vi "clean up vis blockdiagram.vi"(8 "error in (no error)":errorcluster, 10 "Cleanup VI Argument":T3, 11 "Data Cluster in":T1) -> (0 "error out":errorcluster, 2 "Cleanup VI (Reply Payload)":T2, 3 "Data Cluster out":T1)   [LabVIEW 2025, in "Scripting Server.lvlib"]
uses:
  Scripting Server.lvlib
  Cleanup VI Argument--cluster.ctl
  Cleanup VI (Reply Payload)--cluster.ctl
  Module Data--cluster.ctl
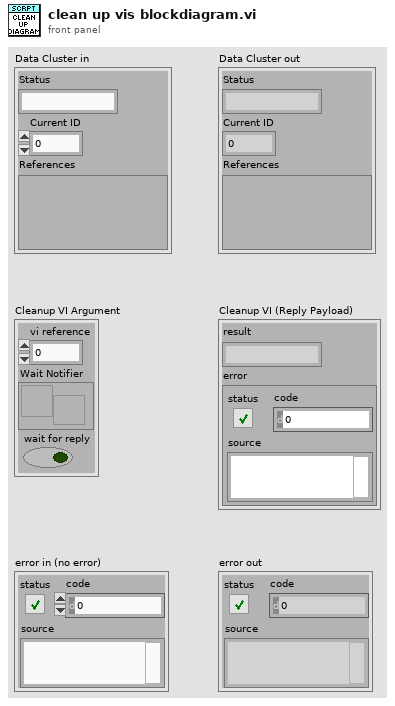
[diagram p1: front panel]
types:
  T1 = typedef "Scripting Server.lvlib/Module Data--cluster.ctl" = cluster{"Status":string, "Current ID":i32, "References":variant}
  T2 = typedef "Scripting Server.lvlib/Cleanup VI (Reply Payload)--cluster.ctl" = cluster{"result":string, "error":errorcluster}
  T3 = typedef "Scripting Server.lvlib/Cleanup VI Argument--cluster.ctl" = cluster{"vi reference":i32, "Wait Notifier":refnum<notifier>, "wait for reply":bool}
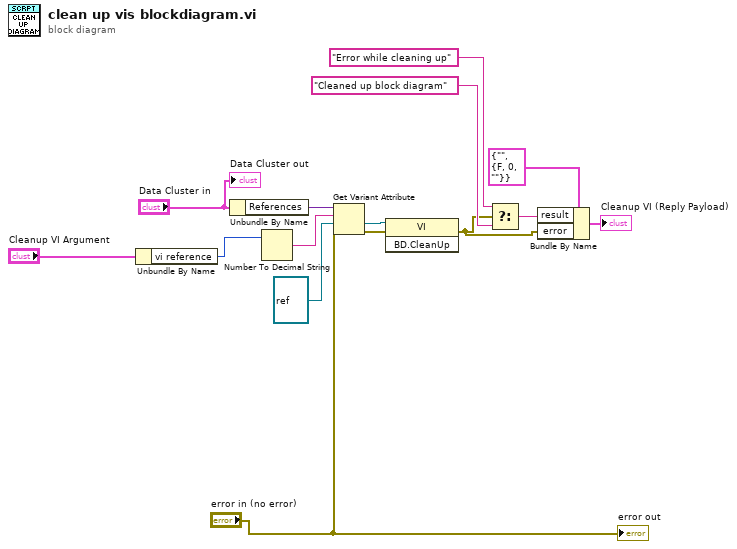
[diagram p0: block diagram]
diagram:
  n1 = Unbundle By Name("Cleanup VI Argument") -> ("vi reference"=w11:i32)
  n2 = Unbundle By Name("Data Cluster in") -> ("References"=w10:variant)
  n3 = Number To Decimal String(number=w11) -> (decimal integer string=w9:string)  [unwired: 1 in]
  n4 = Get Variant Attribute(Variant=w10, name=w9, default value (empty Variant)=refnum<vi> refnum ("vi refnum"), error in="error in (no error)") -> (value=w7:refnum<vi>, error out=w6:errorcluster)  [unwired: 2 out]
  n5 = invoke class="VI" method="BD.CleanUp"(reference=w7, error in=w6) -> (error out=w2:errorcluster)  [unwired: 1 in, 2 out]
  n6 = Select(t="Error while cleaning up" ("result"), s=w2, f="Cleaned up block diagram" ("result")) -> (s? t:f=w3:string)
  n7 = Bundle By Name(cluster=T2 {"result"="", "error"={"status"=FALSE, "code"=0, "source"=""}} ("Cleanup VI (Reply Payload)"), "result"=w3, "error"=w2) -> (→"Cleanup VI (Reply Payload)":T2)
  "Data Cluster out" <- "Data Cluster in"
  "error out" <- "error in (no error)"
